vi "Create.vi"(8 "error in (no error)":errorcluster) -> (0 "error out":errorcluster, 3 "MessageEvent":refnum<user-event>)   [LabVIEW 2019, in "SLL Message.lvlib"]
uses:
  SLL Message.lvlib
  Typedefs/Message.ctl
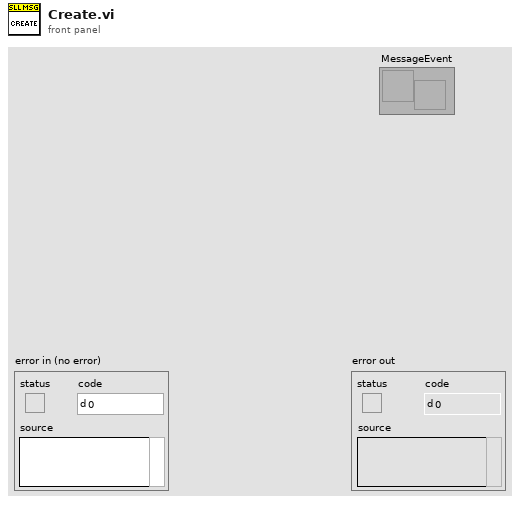
[diagram p1: front panel]
types:
  T1 = typedef "SLL Message.lvlib/Message.ctl" = cluster{"Command":string, "Data":variant, "Fetch Response?":bool, "Response":refnum<notifier>}
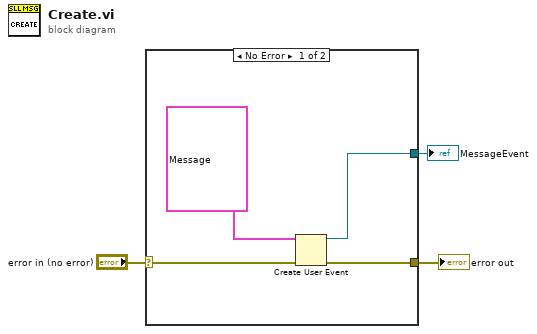
[diagram p0: block diagram]
diagram:
  n1 = case shown="No Error" "error in (no error)" {
    selector: "error in (no error)" -> [w7 w8]
    tunnel: [w6 w8] -> w2
    tunnel: [w4 _] -> w1
    frame No Error {
      n2 = Create User Event(user event datatype=T1 {"Command"="", "Data"=variant, "Fetch Response?"=FALSE, "Response"=refnum} ("Message"), error in=w7) -> (user event=w4:refnum<user-event>, error out=w6:errorcluster)
    }
    frame Error {
    }
  }
  "error out" <- w2
  "MessageEvent" <- w1
